vi "Write to Log File.vi"(8 "error in":errorcluster, 11 "text":string="Log Start") -> (0 "error out":errorcluster)   [LabVIEW 2018, in "Support Library.lvlib" / "Command Logging.lvlib"]
uses:
  Command Logging.lvlib
  File Path.ctl
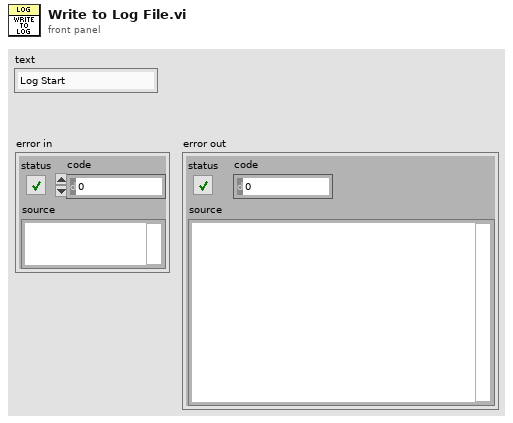
[diagram p1: front panel]
types:
  T1 = typedef "Support Library.lvlib/Command Logging.lvlib/File Path.ctl" = refnum<file>
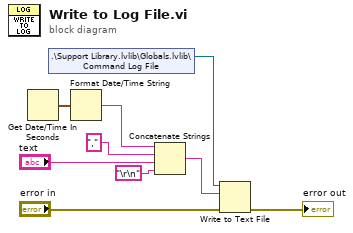
[diagram p0: block diagram]
diagram:
  n1 = Get Date/Time In Seconds() -> (seconds since 1Jan1904=w4:timestamp)
  n2 = shared-variable ".\\Support Library.lvlib\\Globals.lvlib\\Command Log File"() -> (w1:T1)  [unwired: 1 in, 1 out]
  n3 = Format Date/Time String(seconds (now)=w4) -> (date/time string=w3:string)  [unwired: 2 in]
  n4 = Concatenate Strings(w3, "," ("string"), "text", "\r\n") -> (w7:string)
  n5 = Write to Text File(file (use dialog)=w1, text=w7, error in="error in") -> (error out=→"error out":errorcluster)  [unwired: 1 in, 2 out]
